vi "Waveerr.vi"(1 "Numeric":dbl) -> (0 "String":string)   [LabVIEW 2014]
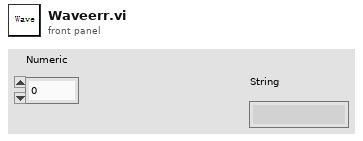
[diagram p1: front panel]
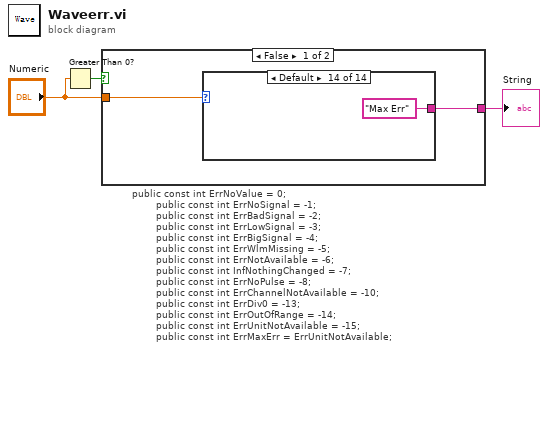
[diagram p0: block diagram]
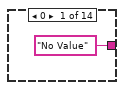
[diagram p2: hidden frame]
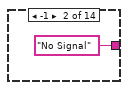
[diagram p3: hidden frame]
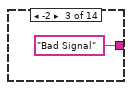
[diagram p4: hidden frame]
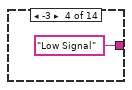
[diagram p5: hidden frame]
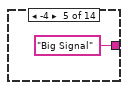
[diagram p6: hidden frame]
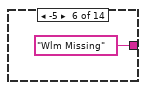
[diagram p7: hidden frame]
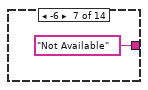
[diagram p8: hidden frame]
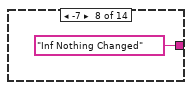
[diagram p9: hidden frame]
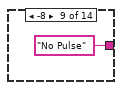
[diagram p10: hidden frame]
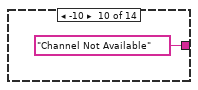
[diagram p11: hidden frame]
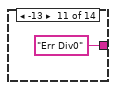
[diagram p12: hidden frame]
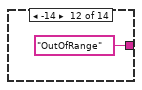
[diagram p13: hidden frame]
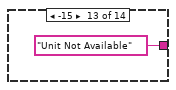
[diagram p14: hidden frame]
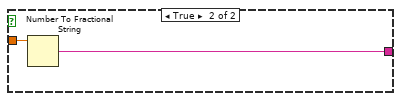
[diagram p15: hidden frame]
diagram:
  # "public const int ErrNoValue = 0;\n        public const int ErrNoSignal = -1;\n        public const int ErrBadSignal = -2;\n        public const int ErrLowSignal = -3;\n        public const int ErrBigSignal = -4;\n        public const int ErrWlmMissing = -5;\n        public const int ErrNotAvailable = -6;\n        public const int InfNothingChanged = -7;\n        public const int ErrNoPulse = -8;\n        public const int ErrChannelNotAvailable = -10;\n        public const int ErrDiv0 = -13;\n        public const int ErrOutOfRange = -14;\n        public const int ErrUnitNotAvailable = -15;\n        public const int ErrMaxErr = ErrUnitNotAvailable;"
  n1 = Greater Than 0?(x="Numeric") -> (x > 0?=w3:bool)
  n2 = case shown="False" w3 {
    tunnel: "Numeric" -> [w5 w21]
    tunnel: [w4 w20] -> w1
    frame False {
      n3 = case shown="Default" w5 {
        tunnel: ["No Value" "No Signal" "Bad Signal" "Low Signal" "Big Signal" "Wlm Missing" "Not Available" "Inf Nothing Changed" "No Pulse" "Channel Not Available" "Err Div0" "OutOfRange" "Unit Not Available" "Max Err"] -> w4
        frame 0 {
        }
        frame -1 {
        }
        frame -2 {
        }
        frame -3 {
        }
        frame -4 {
        }
        frame -5 {
        }
        frame -6 {
        }
        frame -7 {
        }
        frame -8 {
        }
        frame -10 {
        }
        frame -13 {
        }
        frame -14 {
        }
        frame -15 {
        }
        frame Default {
        }
      }
    }
    frame True {
      n4 = Number To Fractional String(number=w21) -> (F-format string=w20:string)  [unwired: 3 in]
    }
  }
  "String" <- w1
